vi "Vacuum Status.vi"() -> (7 "Latched":bool)   [LabVIEW 2014]
panel:
  in  "lower limit: on but not connected":dbl=1.25
  in  "Current threshold":dbl=2.6
  out "current (A)":dbl(knob)=1.125 scale=0.0..6.0
  in  "PDP Channel":i32=8
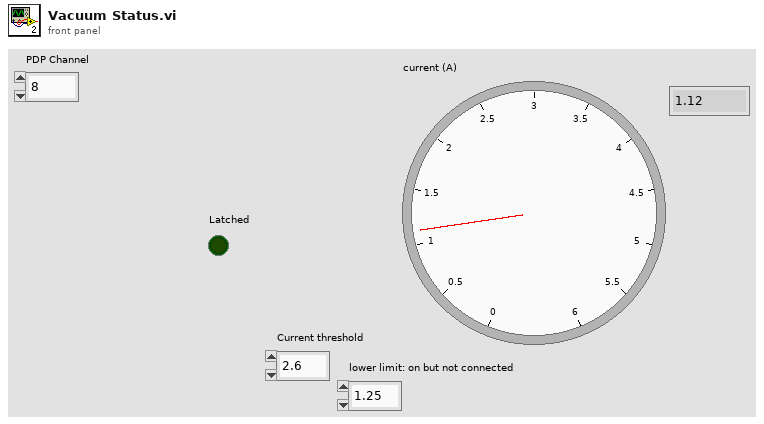
[diagram p1: front panel]
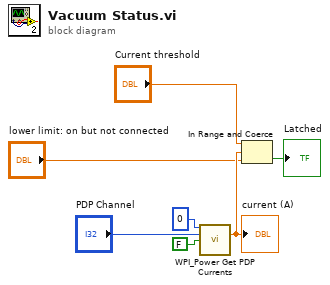
[diagram p0: block diagram]
diagram:
  n1 = call <vilib>:"WPI_Power Get PDP Currents.vi"("Power Distribution Panel (0)"=u8 0, "PDP Channel"="PDP Channel", "Tare Currents?"=FALSE) -> ("current (A)"=w2:dbl)  [unwired: 10 in, 2 out]
  "current (A)" <- w2
  n2 = In Range and Coerce(upper limit="Current threshold", x=w2, lower limit="lower limit: on but not connected") -> (In Range?=→"Latched":bool)  [unwired: 1 out]
